vi "CSM - Get Module Attribute.vi"(0 "CSM Name":string, 5 "Attribute":string, 7 "Default Value (Empty Variant)":variant, 9 "Wait (5000 ms)":i32=5000, 11 "Error In":errorcluster caption="error in (no error)") -> (4 "CSM Name (Dup)":string, 6 "Found":bool, 8 "Value":variant, 10 "Waited (ms)":u32, 15 "error out":errorcluster)   [LabVIEW 2017, in "Communicable State Machine.lvlib"]
doc: "Reads the attribute value of the specified module. If the attribute does not exist, the default value is returned, and <b>Found</b> returns FALSE. Otherwise, it returns TRUE. If the CSM module does not exist, this VI waits for the specified timeout duration. If the timeout is exceeded, this VI returns a timeout error.\n\n\n<b>Reference Example</b>: `[CSM-Example]\\0. Base Concepts\\6. Module Attributes.vi`.\n\n-- <b>Controls</b> --\n- <b>CSM Name</b>: CSM module name.\n- <b>Attribute</b>: Attribute name. Must not be an empty string.\n- <b>Default Value (Empty Variant)</b>: Default value returned when the attribute does not exist.\n- <b>Wait (5000 ms)</b>: Timeout duration for waiting. The default is 5000 ms.\n\n-- <b>Indicators</b> --\n- <b>CSM Name (Dup)</b>: A copy of the input CSM module name.\n- <b>Found</b>: Whether the attribute exists.\n- <b>Value</b>: Attribute value.\n- <b>Waited (ms)</b>: Time elapsed while waiting."
uses:
  Communicable State Machine.lvlib
  _Support/CSMQ/_CSMOFGV(lvlibp).vi
  CSM - Wait for Module to Be Alive.vi
  _Shared/CSM Shared.lvlib
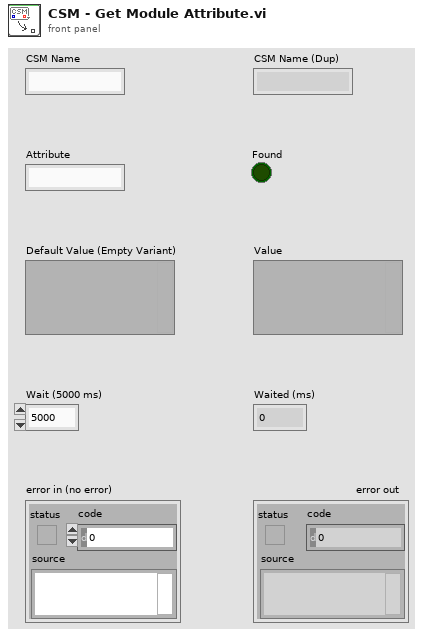
[diagram p1: front panel]
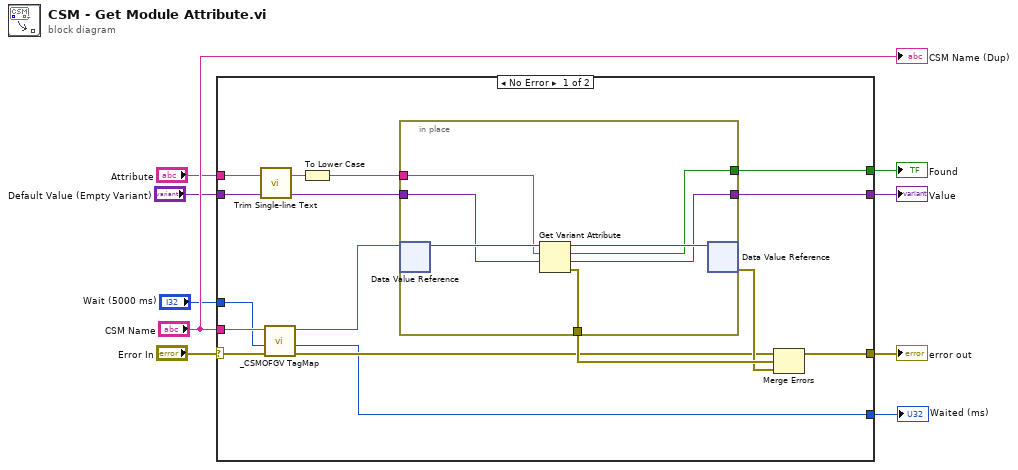
[diagram p0: block diagram]
diagram:
  n1 = case shown="No Error" "Error In" {
    selector: "Error In" -> [w24 w33]
    tunnel: [w21 w33] -> w8
    tunnel: "CSM Name" -> [w16 _]
    tunnel: "Attribute" -> [w11 _]
    tunnel: "Default Value (Empty Variant)" -> [w20 w32]
    tunnel: [w19 _] -> w4
    tunnel: [w18 w32] -> w3
    tunnel: [w15 _] -> w2
    tunnel: "Wait (5000 ms)" -> [w14 _]
    frame No Error {
      n2 = call "Trim Single-line Text.vi"("single-line text"=w11) -> ("trimed text"=w12:string)  [unwired: 2 in]
      n3 = call "_CSMOFGV TagMap.vi"("error in (no error)"=w24, "Wait (5000 ms)"=w14, "CSM Name"=w16) -> ("error out"=w17:errorcluster, "Waited (ms)"=w15:u32, "TagMap"=w13:refnum<data-value>)  [unwired: 6 in]
      n4 = To Lower Case(string=w12) -> (all lower case string=w10:string)
      n5 = in-place {
        in-place-border: [w29] -> w23
        in-place-border: w10 -> [w28]
        in-place-border: w20 -> [w27]
        in-place-border: [w26] -> w19
        in-place-border: [w25] -> w18
        n6 = in-place-dvr #1(w13) -> (w31:variant)  [unwired: 1 out]
        n7 = Get Variant Attribute(Variant=w31, name=w28, default value (empty Variant)=w27) -> (duplicate Variant=w30:variant, found=w26:bool, value=w25:variant, error out=w29:errorcluster)  [unwired: 1 in]
        n8 = in-place-dvr #1(w30) -> (w22:errorcluster)  [unwired: 1 out]
      }
      n9 = Merge Errors(w17, w23, w22) -> (w21:errorcluster)
    }
    frame Error {
    }
  }
  "error out" <- w8
  "Value" <- w3
  "Found" <- w4
  "Waited (ms)" <- w2
  "CSM Name (Dup)" <- "CSM Name"
